vi "AOIcut.vi"(7 "AOI":cluster{"AOI h, px":dbl, "AOI w, px":dbl}, 11 "image data in":T1) -> (3 "image data out":T1)   [LabVIEW 2017]
uses:
  <vilib>/picture/picture.llb/imagedata.ctl
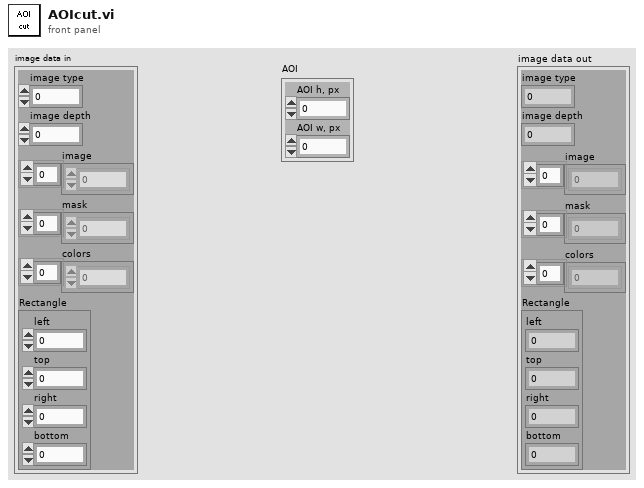
[diagram p1: front panel]
types:
  T1 = typedef "imagedata.ctl" = cluster{"image type":i32, "image depth":i32, "image":u8[], "mask":u8[], "colors":u32[], "Rectangle":cluster{"left":i16, "top":i16, "right":i16, "bottom":i16}}
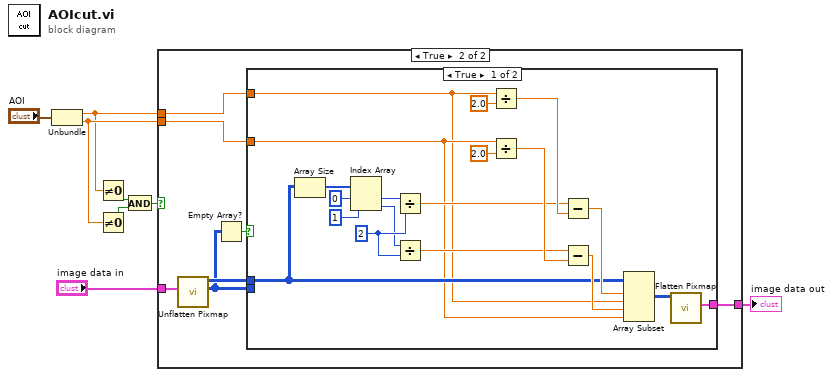
[diagram p0: block diagram]
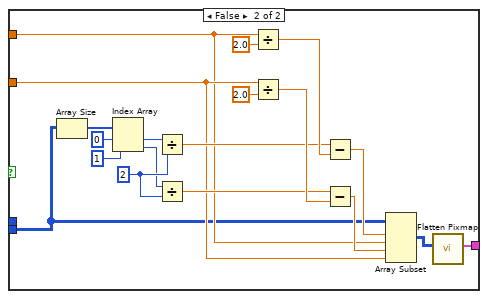
[diagram p3: hidden frame]
diagram:
  n1 = Unbundle("AOI") -> ("AOI h, px"=w4:dbl, "AOI w, px"=w5:dbl)
  n2 = Not Equal To 0?(x=w4) -> (x != 0?=w3:bool)
  n3 = Not Equal To 0?(x=w5) -> (x != 0?=w2:bool)
  n4 = And(x=w3, y=w2) -> (x .and. y?=w1:bool)
  n5 = case shown="True" w1 {
    tunnel: [w9 w16] -> w8
    tunnel: "image data in" -> [w9 w15]
    tunnel: w5 -> [_ w12]
    tunnel: w4 -> [_ w11]
    frame False {
    }
    frame True {
      n6 = call <vilib>:"Unflatten Pixmap.vi"("image data"=w15) -> ("8-bit pixmap"=w13:u8[][], "24-bit pixmap"=w14:u32[][])  [unwired: 4 in, 5 out]
      n7 = Empty Array?(array=w13) -> (empty?=w10:bool)
      n8 = case shown="True" w10 {
        tunnel: [w35 w54] -> w16
        tunnel: w14 -> [w19 _]
        tunnel: w12 -> [w18 w39]
        tunnel: w11 -> [w17 w38]
        tunnel: w13 -> [_ w37]
        frame True {
          w25 = 2 ("y")
          n9 = Array Size(array=w19) -> (size(s)=w20:i32[])
          n10 = Index Array(array=w20, index #1=0 ("index"), index #2=1 ("index")) -> (element #1=w23:i32, element #2=w24:i32)
          n11 = Divide(x=w23, y=w25) -> (x/y=w26:dbl)
          n12 = Divide(x=w24, y=w25) -> (x/y=w27:dbl)
          n13 = Divide(x=w17, y=2.0) -> (x/y=w33:dbl)
          n14 = Divide(x=w18, y=2.0) -> (x/y=w32:dbl)
          n15 = Subtract(x=w26, y=w33) -> (x-y=w29:dbl)
          n16 = Subtract(x=w27, y=w32) -> (x-y=w28:dbl)
          n17 = Array Subset(array=w19, index (row)=w29, length (row)=w17, index (col)=w28, length (col)=w18) -> (w34:u32[][])
          n18 = call <vilib>:"Flatten Pixmap.vi"("24-bit pixmap"=w34) -> ("image data"=w35:T1)  [unwired: 10 in]
        }
        frame False {
          w45 = 2 ("y")
          n19 = Array Size(array=w37) -> (size(s)=w40:i32[])
          n20 = Index Array(array=w40, index #1=0 ("index"), index #2=1 ("index")) -> (element #1=w43:i32, element #2=w44:i32)
          n21 = Divide(x=w43, y=w45) -> (x/y=w46:dbl)
          n22 = Divide(x=w44, y=w45) -> (x/y=w47:dbl)
          n23 = Divide(x=w38, y=2.0) -> (x/y=w53:dbl)
          n24 = Divide(x=w39, y=2.0) -> (x/y=w52:dbl)
          n25 = Subtract(x=w46, y=w53) -> (x-y=w49:dbl)
          n26 = Subtract(x=w47, y=w52) -> (x-y=w48:dbl)
          n27 = Array Subset(array=w37, index (row)=w49, length (row)=w38, index (col)=w48, length (col)=w39) -> (w36:u8[][])
          n28 = call <vilib>:"Flatten Pixmap.vi"("8-bit pixmap"=w36) -> ("image data"=w54:T1)  [unwired: 10 in]
        }
      }
    }
  }
  "image data out" <- w8
